vi "Set DO Status - All.vi"(0 "reference in":refnum<class "DO.lvclass">, 4 "All DO On/Off":bool, 5 "error in (no error)":errorcluster) -> (14 "reference out":refnum<class "DO.lvclass">, 19 "error out":errorcluster)   [LabVIEW 2017, in "DO.lvclass"]
uses:
  DO.lvclass
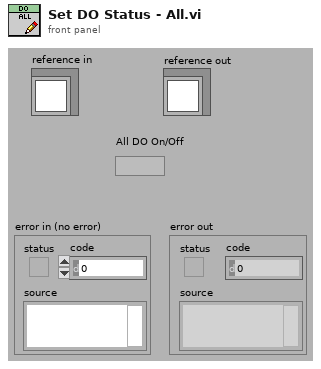
[diagram p1: front panel]
types:
  T1 = typedef "DO.lvclass/ObjectAttributes.ctl" = cluster{"DO Task":refnum<k21>, "DO Module Names (NI-Max Name)":string[], "Number of Channels Per DO Module":i32[], "DO Status":bool[], "Number of DO Modules":u32, "DO Status to Set":bool[], "DO On/Off Status":bool, "DO VI Reference":refnum<vi>, "Number of Total DO Channels":u32}
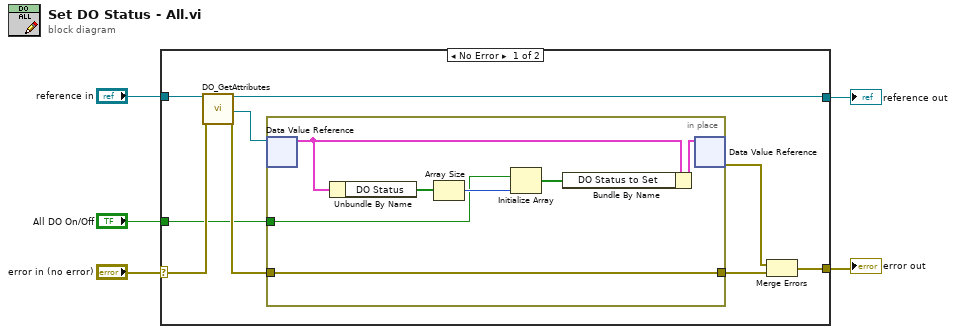
[diagram p0: block diagram]
diagram:
  n1 = case shown="No Error" "error in (no error)" {
    selector: "error in (no error)" -> [w13 w23]
    tunnel: [w10 w23] -> w4
    tunnel: [w11 w22] -> w2
    tunnel: "reference in" -> [w14 w22]
    tunnel: "All DO On/Off" -> [w6 _]
    frame No Error {
      n2 = call "DO_GetAttributes.vi"("reference in"=w14, "error in (no error)"=w13) -> ("reference out"=w11:refnum<class "DO.lvclass">, "DataRef"=w9:refnum<data-value>, "error out"=w8:errorcluster)  [unwired: 14 in, 1 out]
      n3 = in-place {
        in-place-border: w8 -> [w19]
        in-place-border: [w19] -> w7
        in-place-border: w6 -> [w16]
        n4 = in-place-dvr #1(w9) -> (w20:T1)  [unwired: 1 out]
        n5 = Unbundle By Name(w20) -> ("DO Status"=w17:bool[])
        n6 = Array Size(array=w17) -> (size(s)=w18:i32)
        n7 = Initialize Array(w16, w18) -> (w15:bool[])
        n8 = Bundle By Name(cluster=w20, "DO Status to Set"=w15) -> (w21:T1)
        n9 = in-place-dvr #1(w21) -> (w12:errorcluster)  [unwired: 1 out]
      }
      n10 = Merge Errors(w12, w7) -> (w10:errorcluster)
    }
    frame Error {
    }
  }
  "error out" <- w4
  "reference out" <- w2
